vi "URAPI_WhileEnd.vi"(3 "URAPI Script":T1={"Script"="", "Whiles"=[], "Ifs"=[], "Supress Err"=TRUE, "Errors"=""}) -> (5 "URAPI Script Out":T1={"Script"="", "Whiles"=[], "Ifs"=[], "Supress Err"=TRUE, "Errors"=""})   [LabVIEW 2012]
doc: "Causes a script loop to iterate. Required by both while and for loops."
uses:
  <userlib>/BotSpeak/VIs/Direct/URAPI_Control.ctl
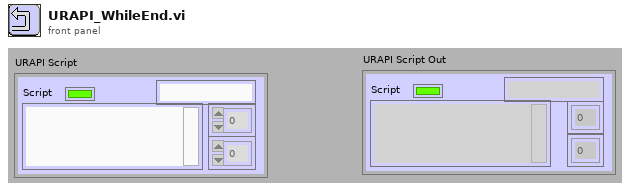
[diagram p1: front panel]
types:
  T1 = typedef "URAPI_Control.ctl" = cluster{"Script":string, "Whiles":u8[], "Ifs":u8[], "Supress Err":bool, "Errors":string}
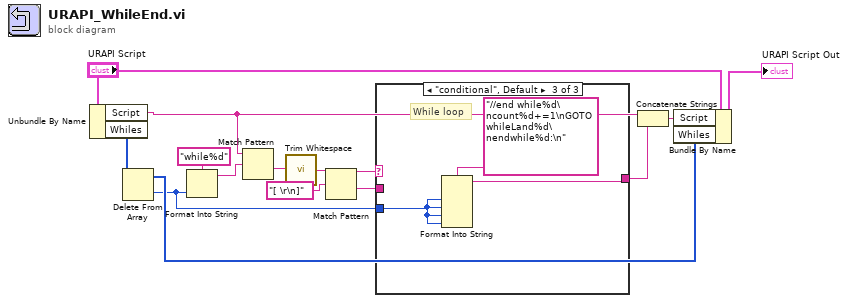
[diagram p0: block diagram]
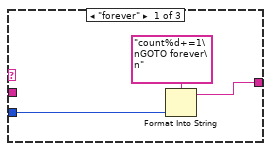
[diagram p2: hidden frame]
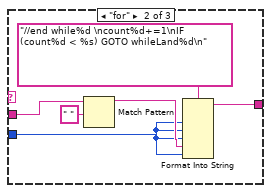
[diagram p3: hidden frame]
diagram:
  n1 = Unbundle By Name("URAPI Script") -> ("Script"=w7:string, "Whiles"=w11:u8[])
  n2 = Delete From Array(array=w11) -> (deleted portion=w6:u8, array with subset deleted=w10:u8[])  [unwired: 2 in]
  n3 = Format Into String(format string="while%d" ("string"), w6) -> (resulting string=w8:string)  [unwired: 2 in, 1 out]
  n4 = Match Pattern(string=w7, regular expression=w8) -> (after substring=w5:string)  [unwired: 1 in, 3 out]
  n5 = call <vilib>:"Trim Whitespace.vi"("string"=w5) -> ("trimmed string"=w4:string)  [unwired: 1 in]
  n6 = Match Pattern(string=w4, regular expression="[ \r\n]") -> (before substring=w2:string, after substring=w1:string)  [unwired: 1 in, 2 out]
  n7 = case shown="\"conditional\", Default" w2 {
    tunnel: [w16 w23 w26] -> w12
    tunnel: w6 -> [w17 w19 w25]
    tunnel: w1 -> [_ w20 _]
    frame "forever" {
      n8 = Format Into String(format string="count%d+=1\nGOTO forever\n", w17) -> (resulting string=w16:string)  [unwired: 2 in, 1 out]
    }
    frame "for" {
      n9 = Match Pattern(string=w20, regular expression=" ") -> (before substring=w21:string)  [unwired: 1 in, 3 out]
      n10 = Format Into String(format string="//end while%d \ncount%d+=1\nIF (count%d < %s) GOTO whileLand%d\n" ("string"), w19, w19, w19, w21, w19) -> (resulting string=w23:string)  [unwired: 2 in, 1 out]
    }
    frame "conditional", Default {
      # "While loop"
      n11 = Format Into String(format string="//end while%d\ncount%d+=1\nGOTO whileLand%d\nendwhile%d:\n" ("string"), w25, w25, w25, w25) -> (resulting string=w26:string)  [unwired: 2 in, 1 out]
    }
  }
  n12 = Concatenate Strings(w7, w12) -> (w14:string)
  n13 = Bundle By Name(cluster="URAPI Script", "Script"=w14, "Whiles"=w10) -> (→"URAPI Script Out":T1)
